vi "Send TCP Data.vi"(0 "connection ID":refnum<k5>, 1 "Data in":dbl[][](array[numeric]), 3 "error in (no error)":errorcluster, 4 "Single precision?":bool=TRUE) -> (7 "connection ID 2":refnum<k5>, 10 "error out":errorcluster)   [LabVIEW 2015]
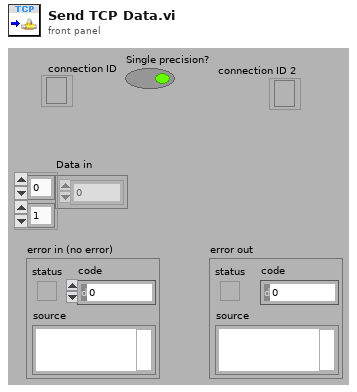
[diagram p1: front panel]
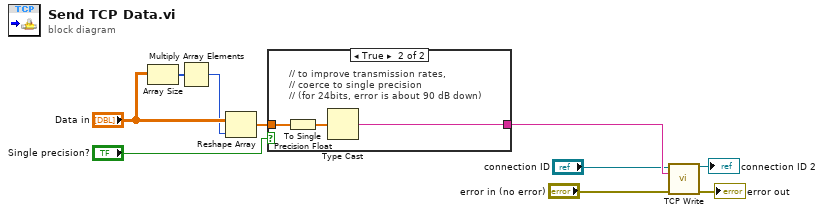
[diagram p0: block diagram]
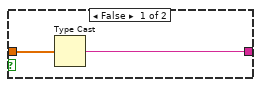
[diagram p2: hidden frame]
diagram:
  n1 = Array Size(array="Data in") -> (size(s)=w10:i32[])
  n2 = Multiply Array Elements(1:w10) -> (0:w6:i32)
  n3 = Reshape Array("Data in", w6) -> (w8:dbl[])
  n4 = case shown="True" "Single precision?" {
    tunnel: w8 -> [w12 w15]
    tunnel: [w11 w13] -> w5
    frame False {
      n5 = Type Cast(x=w12) -> (*(type *) &x=w11:string)  [unwired: 1 in]
    }
    frame True {
      # "// to improve transmission rates,\n// coerce to single precision\n// (for 24bits, error is about 90 dB down)"
      n6 = To Single Precision Float(number=w15) -> (single precision float=w14:sgl[])
      n7 = Type Cast(x=w14) -> (*(type *) &x=w13:string)  [unwired: 1 in]
    }
  }
  n8 = call "TCP Write.vi"("connection ID"="connection ID", "data string"=w5, "error in (no error)"="error in (no error)") -> ("connection ID out"=→"connection ID 2":refnum<k5>, "error out"=→"error out":errorcluster)  [unwired: 10 in, 1 out]
